vi "DUAL GAUGE-Test Display,IO.vi"(8 "Fehler (Eingang)":errorcluster, 9 "Testfunction":u8(ring) items=["Display Test", "I/O Test"], 11 "Referenz in":refnum<visa-resource-name>) -> (0 "Cluster (Ausgang)":errorcluster, 3 "Referenz out":refnum<visa-resource-name>)   [LabVIEW 2010, in "Dual Gauge.lvlib"]
uses:
  Dual Gauge.lvlib
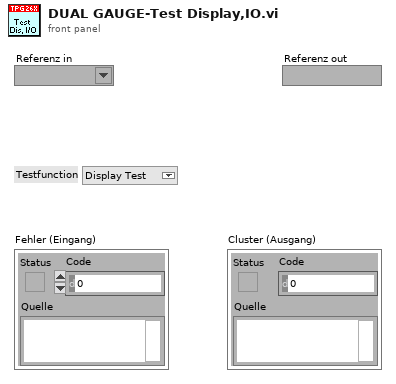
[diagram p1: front panel]
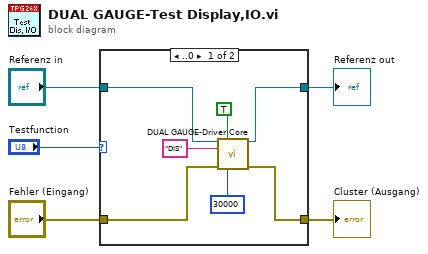
[diagram p0: block diagram]
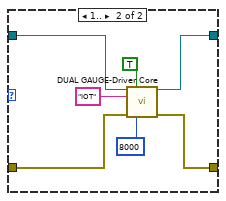
[diagram p2: hidden frame]
diagram:
  n1 = case shown="..0" "Testfunction" {
    tunnel: [w10 w18] -> w4
    tunnel: "Referenz in" -> [w8 w15]
    tunnel: "Fehler (Eingang)" -> [w6 w14]
    tunnel: [w7 w13] -> w1
    frame ..0 {
      n2 = call "DUAL GAUGE-Driver Core.vi"("Referenz in"=w8, "Write/Read"=TRUE, "Command"="DIS", "Fehler (Eingang)"=w6, "Timeout [ms]"=u32 30000) -> ("Referenz out"=w7:refnum<visa-resource-name>, "Cluster (Ausgang)"=w10:errorcluster)  [unwired: 8 in, 1 out]
    }
    frame 1.. {
      n3 = call "DUAL GAUGE-Driver Core.vi"("Referenz in"=w15, "Write/Read"=TRUE, "Command"="IOT", "Fehler (Eingang)"=w14, "Timeout [ms]"=u32 8000) -> ("Referenz out"=w13:refnum<visa-resource-name>, "Cluster (Ausgang)"=w18:errorcluster)  [unwired: 8 in, 1 out]
    }
  }
  "Cluster (Ausgang)" <- w4
  "Referenz out" <- w1
